vi "WaveGeneratorSetup.vi"(6 "Frequency":u16, 7 "stimulus specifier":T3, 8 "Stimulus\nduration (s)":dbl, 9 "Time between stimuli,\nstart-to-start (s)":dbl, 10 "Number\nof stimuli":u16, 11 "Initial delay (s)":dbl) -> (0 "error IO":errorcluster, 1 "stimulus parameters":T1, 2 "stimulus information":T2, 3 "stimulus specifier":T3)   [LabVIEW 2014]
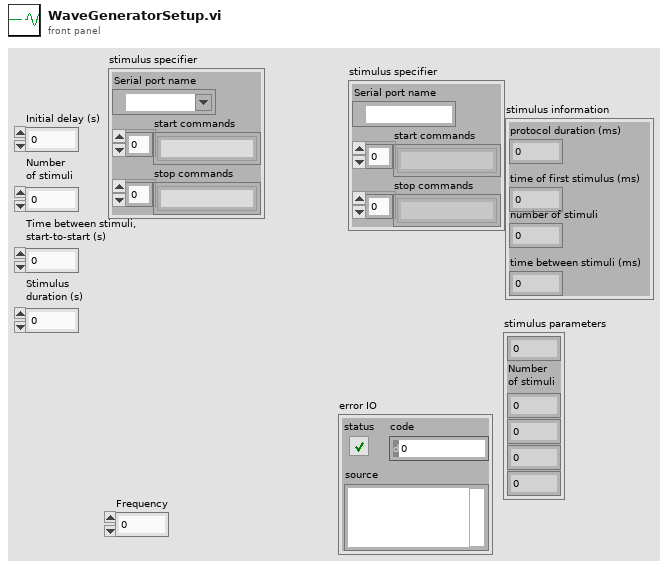
[diagram p1: front panel]
types:
  T1 = cluster{dbl, "Number\nof stimuli":u16, dbl, dbl, u16}
  T2 = cluster{"protocol duration (ms)":i64, "time of first stimulus (ms)":i64, "number of stimuli":u16, "time between stimuli (ms)":i64}
  T3 = cluster{"Serial port name":refnum<visa-resource-name>, "start commands":string[], "stop commands":string[]}
  T4 = cluster{i64, "result (ms)":i64, "Number\nof stimuli":u16, i64}
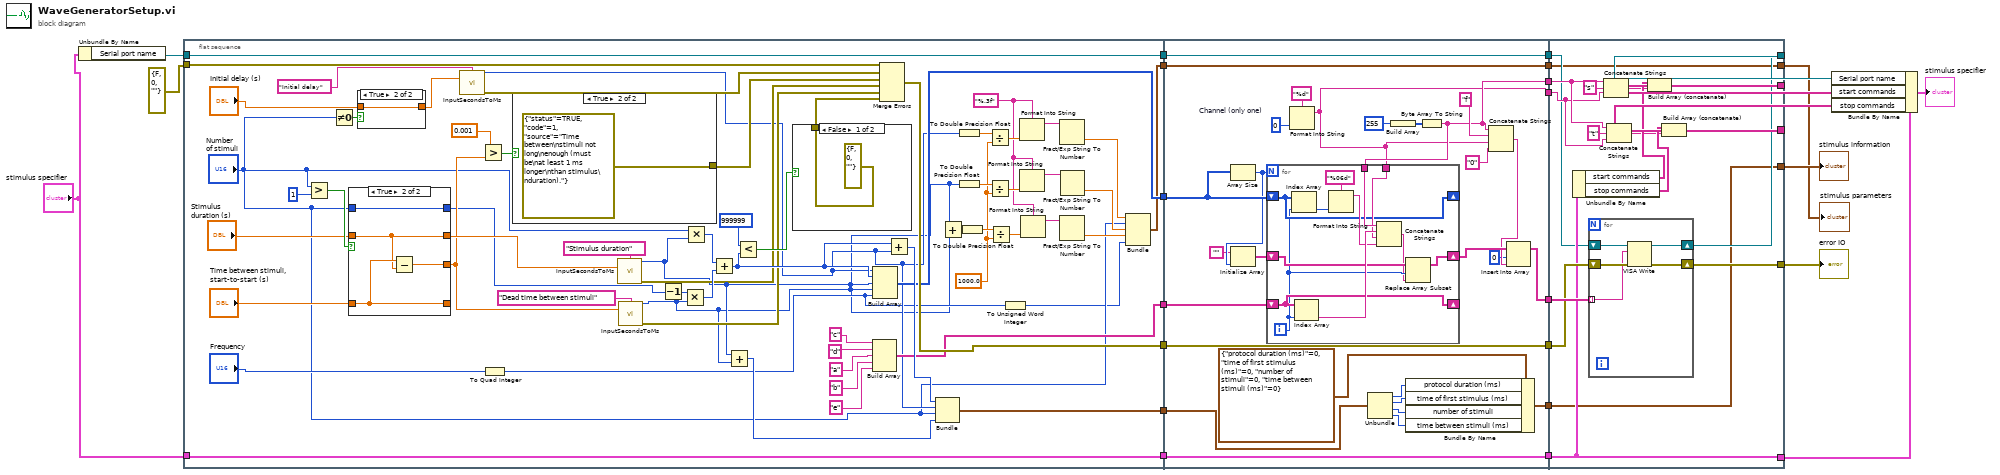
[diagram p0: block diagram]
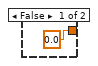
[diagram p2: hidden frame]
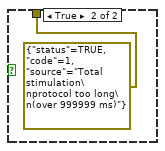
[diagram p3: hidden frame]
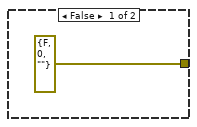
[diagram p4: hidden frame]
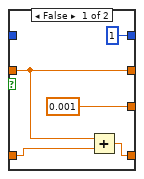
[diagram p5: hidden frame]
diagram:
  n1 = Unbundle By Name("stimulus specifier") -> ("Serial port name"=w12:refnum<visa-resource-name>)
  n2 = flat-sequence {
    tunnel: [w50] -> w9
    tunnel: [w49] -> w8
    tunnel: [w67] -> w7
    tunnel: [w65] -> w6
    tunnel: [w62] -> w5
    tunnel: "stimulus specifier" -> [w65]
    tunnel: errorcluster {"status"=FALSE, "code"=0, "source"=""} ("error constant") -> [w57]
    tunnel: w12 -> [w56]
    tunnel: [w56] -> w4
    tunnel: [w27] -> w3
    tunnel: w9 -> [w132]
    tunnel: w8 -> [w131]
    tunnel: w7 -> [w118]
    tunnel: [w119] -> w26
    tunnel: [w118] -> w25
    tunnel: [w117] -> w24
    tunnel: [w116] -> w23
    tunnel: w6 -> [w115]
    tunnel: [w115] -> w21
    tunnel: w5 -> [w113]
    tunnel: [w108] -> w15
    tunnel: w4 -> [w107]
    tunnel: [w107] -> w11
    tunnel: w3 -> [w105]
    tunnel: [w105] -> w2
    tunnel: w26 -> [w162]
    tunnel: w25 -> [w161]
    tunnel: w24 -> [w158]
    tunnel: w23 -> [w157]
    tunnel: [w156] -> w22
    tunnel: w21 -> [w148]
    tunnel: [w155] -> w19
    tunnel: [w150] -> w18
    tunnel: [w149] -> w17
    tunnel: [w148] -> w20
    tunnel: w15 -> [w147]
    tunnel: [w147] -> w14
    tunnel: w11 -> [w146]
    tunnel: w2 -> [w145]
    tunnel: [w145] -> w1
    frame #0 {
      w39 = 1000.0 ("default (0 I32)")
      w38 = "%.3f"
      n3 = Greater?(x="Number\nof stimuli", y=u16 1) -> (0:w88:bool)
      n4 = Not Equal To 0?(x="Number\nof stimuli") -> (x != 0?=w60:bool)
      n5 = case shown="True" w88 {
        tunnel: "Time between stimuli,\nstart-to-start (s)" -> [w98 w103]
        tunnel: [w99 w103] -> _
        tunnel: "Number\nof stimuli" -> [_ w104]
        tunnel: "Stimulus\nduration (s)" -> [w97 w102]
        tunnel: [w97 w102] -> w82
        tunnel: [u16 1 ("Number\nof stimuli") w104] -> w77
        tunnel: [0.001 w101] -> w80
        frame False {
          n6 = Add(x=w97, y=w98) -> (x+y=w99:dbl)
        }
        frame True {
          n7 = Subtract(x=w103, y=w102) -> (x-y=w101:dbl)
        }
      }
      n8 = case shown="True" w60 {
        tunnel: "Initial delay (s)" -> [_ w91]
        tunnel: [0.0 ("Initial delay (s)") w91] -> w58
        frame False {
        }
        frame True {
        }
      }
      n9 = call "InputSecondsToMs.vi"("description"="Initial delay", "value (s)"=w58) -> ("result (ms)"=w33:i64, "error out"=w85:errorcluster)  [unwired: 12 in]
      n10 = Greater?(x=0.001, y=w80) -> (0:w55:bool)
      n11 = To Quad Integer(1:"Frequency") -> (0:w31:i64)
      n12 = case shown="True" w55 {
        tunnel: [errorcluster {"status"=FALSE, "code"=0, "source"=""} ("error constant") errorcluster {"status"=TRUE, "code"=1, "source"="Time between\nstimuli not long\nenough (must be\nat least 1 ms longer\nthan stimulus\nduration)."} ("error constant")] -> w83
        frame False {
        }
        frame True {
        }
      }
      n13 = call "InputSecondsToMs.vi"("description"="Stimulus duration", "value (s)"=w82) -> ("result (ms)"=w29:i64, "error out"=w53:errorcluster)  [unwired: 12 in]
      n14 = call "InputSecondsToMs.vi"("description"="Dead time between stimuli", "value (s)"=w80) -> ("result (ms)"=w28:i64, "error out"=w52:errorcluster)  [unwired: 12 in]
      n15 = Decrement(x=w77) -> (x-1=w78:u16)
      n16 = Multiply(x=w78, y=w28) -> (x*y=w75:i64)
      n17 = Multiply(x="Number\nof stimuli", y=w29) -> (x*y=w76:i64)
      n18 = Add(x=w76, y=w75) -> (x+y=w66:i64)
      n19 = Add(x=w29, y=w28) -> (x+y=w64:i64)
      n20 = Less?(x=i64 999999, y=w66) -> (x < y?=w73:bool)
      n21 = case shown="False" w73 {
        tunnel: [errorcluster {"status"=FALSE, "code"=0, "source"=""} ("error constant") errorcluster {"status"=TRUE, "code"=1, "source"="Total stimulation\nprotocol too long\n(over 999999 ms)"} ("error constant")] -> w51
        frame False {
        }
        frame True {
        }
      }
      n22 = Build Array("c" ("description"), "d" ("description"), "a" ("description"), "b" ("description"), "e" ("description")) -> (w49:string[])
      n23 = Build Array(w33, w66, w29, w28, w31) -> (w50:i64[])
      n24 = Merge Errors(w57, w85, w83, w53, w52, w51) -> (w67:errorcluster)
      n25 = Add(x=w66, y=w33) -> (x+y=w63:i64)
      n26 = Bundle(w63, "result (ms)"=w33, "Number\nof stimuli"="Number\nof stimuli", w64) -> (w62:T4)  [unwired: 1 in]
      n27 = Add(x=w29, y=w28) -> (x+y=w35:i64)
      n28 = To Double Precision Float(number=w33) -> (double precision float=w46:dbl)
      n29 = To Double Precision Float(number=w29) -> (double precision float=w43:dbl)
      n30 = To Double Precision Float(number=w35) -> (double precision float=w40:dbl)
      n31 = Divide(x=w46, y=w39) -> (x/y=w47:dbl)
      n32 = Divide(x=w43, y=w39) -> (x/y=w44:dbl)
      n33 = Divide(x=w40, y=w39) -> (x/y=w41:dbl)
      n34 = To Unsigned Word Integer(number=w31) -> (unsigned 16bit integer=w30:u16)
      n35 = Format Into String(format string=w38, w47) -> (resulting string=w48:string)  [unwired: 2 in, 1 out]
      n36 = Format Into String(format string=w38, w44) -> (resulting string=w45:string)  [unwired: 2 in, 1 out]
      n37 = Format Into String(format string=w38, w41) -> (resulting string=w42:string)  [unwired: 2 in, 1 out]
      n38 = Fract/Exp String To Number(string=w48) -> (number=w37:dbl)  [unwired: 3 in, 1 out]
      n39 = Fract/Exp String To Number(string=w42) -> (number=w34:dbl)  [unwired: 3 in, 1 out]
      n40 = Fract/Exp String To Number(string=w45) -> (number=w36:dbl)  [unwired: 3 in, 1 out]
      n41 = Bundle(w37, "Number\nof stimuli"="Number\nof stimuli", w36, w34, w30) -> (w27:T1)  [unwired: 1 in]
    }
    frame #1 {
      w106 = i16 0  # Channel (only one)
      n42 = Array Size(array=w132) -> (size(s)=w127:i32)
      n43 = Initialize Array("", w127) -> (w125:string[])
      n44 = Format Into String(format string="%d", w106) -> (resulting string=w116:string)  [unwired: 2 in, 1 out]
      n45 = Unbundle(w113) -> (w112:i64, "result (ms)"=w111:i64, "Number\nof stimuli"=w110:u16, w109:i64)
      n46 = Build Array(u8 255 ("element")) -> (w129:u8[])
      n47 = Bundle By Name(cluster=T2 {"protocol duration (ms)"=0, "time of first stimulus (ms)"=0, "number of stimuli"=0, "time between stimuli (ms)"=0}, "protocol duration (ms)"=w112, "time of first stimulus (ms)"=w111, "number of stimuli"=w110, "time between stimuli (ms)"=w109) -> (w108:T2)
      n48 = Byte Array To String(unsigned byte array=w129) -> (string=w117:string)
      n49 = for {
        N: w127 -> [_]
        shift-right: [w137] -> _
        shift-left: w132 -> [w137]
        shift-right: [w138] -> _
        shift-left: w131 -> [w138]
        tunnel: w117 -> [w142]
        tunnel: w116 -> [w140]
        shift-right: [w136] -> w124
        shift-left: w125 -> [w135]
        i -> [w134]
        n50 = Index Array(array=w137, index=w134) -> (element=w144:i64)
        n51 = Index Array(array=w138, index=w134) -> (element=w141:string)
        n52 = Format Into String(format string="%06d", w144) -> (resulting string=w139:string)  [unwired: 2 in, 1 out]
        n53 = Concatenate Strings(w142, w141, w140, w139) -> (w133:string)
        n54 = Replace Array Subset(array=w135, new element=w133, index=w134) -> (w136:string[])
      }
      n55 = Concatenate Strings(w117, "f" ("string"), w116, "0" ("string")) -> (w121:string)
      n56 = Insert Into Array(array=w124, index=0, new element=w121) -> (w119:string[])
    }
    frame #2 {
      n57 = Unbundle By Name(w148) -> ("start commands"=w154:string[], "stop commands"=w152:string[])
      n58 = for {
        tunnel: w162 -> [w163] mode=indexing
        shift-right: [w166] -> w155
        shift-left: w146 -> [w167]
        shift-right: [w164] -> w156
        shift-left: w161 -> [w165]
        n59 = VISA Write(VISA resource name=w167, write buffer=w163, error in (no error)=w165) -> (VISA resource name out=w166:refnum<visa-resource-name>, error out=w164:errorcluster)  [unwired: 1 out]
      }
      n60 = Concatenate Strings(w158, "s" ("string"), w157) -> (w153:string)
      n61 = Concatenate Strings(w158, "t" ("string"), w157) -> (w151:string)
      n62 = Build Array (concatenate)(w154, w153) -> (w150:string[])
      n63 = Build Array (concatenate)(w152, w151) -> (w149:string[])
    }
  }
  n64 = Bundle By Name(cluster=w20, "Serial port name"=w19, "start commands"=w18, "stop commands"=w17) -> (→"stimulus specifier":T3)
  "error IO" <- w22
  "stimulus information" <- w14
  "stimulus parameters" <- w1
